vi "Program Ramp.vi"(8 "error in (no error)":errorcluster, 9 "Ramp rate, K/min":dbl=1.0, 10 "Approach":T1, 11 "LakeShore T Controller in":refnum<class "LakeShore T Controller.lvclass">) -> (0 "error out":errorcluster, 3 "LakeShore T Controller out":refnum<class "LakeShore T Controller.lvclass">)   [LabVIEW 2015, in "LakeShore T Controller.lvclass"]
uses:
  LakeShore T Controller.lvclass
  Instruments/Neocera/Neocera Set Point Aproach.ctl
  Mag Lab Hardware.lvclass/Mag Lab Hardware.ctl
  Mag Lab Hardware.lvclass
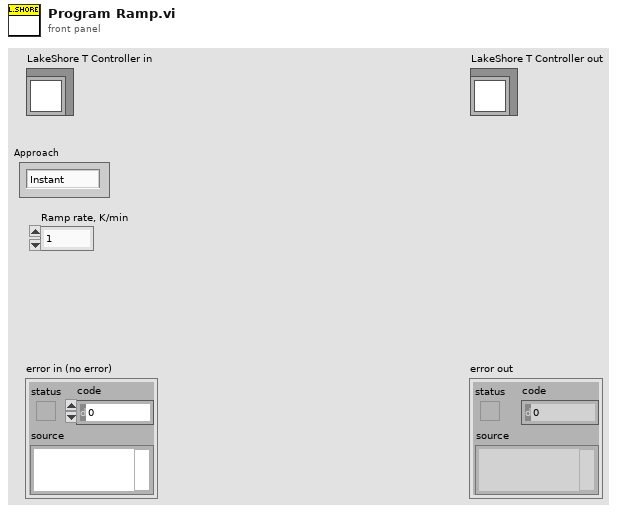
[diagram p1: front panel]
types:
  T1 = typedef "Neocera Set Point Aproach.ctl" = enum16{"Instant", "Ramp"}
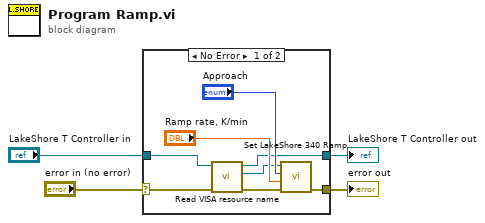
[diagram p0: block diagram]
diagram:
  n1 = case shown="No Error" "error in (no error)" {
    selector: "error in (no error)" -> [w6 w14]
    tunnel: [w5 w14] -> w3
    tunnel: [w9 w13] -> w1
    tunnel: "LakeShore T Controller in" -> [w12 w13]
    frame No Error {
      n2 = call "Read VISA resource name.vi"("error in (no error)"=w6, "Mag Lab Hardware in"=w12) -> ("error out"=w7:errorcluster, "VISA resource name"=w8:refnum<visa-resource-name>, "Mag Lab Hardware out"=w9:refnum<class "LakeShore T Controller.lvclass">)  [unwired: 7 in]
      n3 = call "Set LakeShore 340 Ramp.vi"("error in (no error)"=w7, "Ramp rate, K/min"="Ramp rate, K/min", "Approach"="Approach", "VISA resource name"=w8) -> ("error out"=w5:errorcluster)  [unwired: 6 in, 1 out]
    }
    frame Error {
    }
  }
  "error out" <- w3
  "LakeShore T Controller out" <- w1
